vi "read.vi"() -> ()   [LabVIEW 2020]
panel:
  in  "lim 2":dbl
  in  "Temp":dbl(slide) scale=0.0..100.0
  out "Waveform Chart":dynamicdata(graph)
  in  "stop":bool
  out "alarma":bool
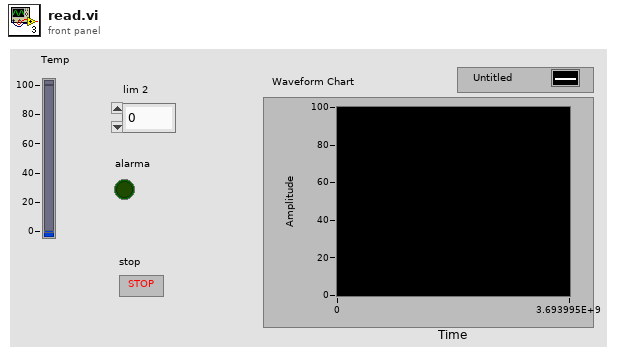
[diagram p1: front panel]
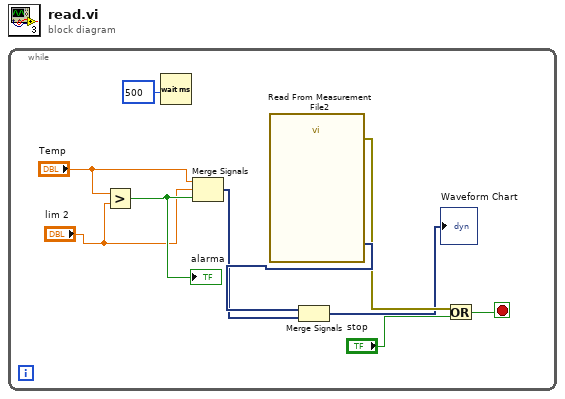
[diagram p0: block diagram]
diagram:
  n1 = while {
    stop <- w9 stop-if-true
    n2 = Greater?(x="Temp", y="lim 2") -> (0:w5:bool)
    "alarma" <- w5
    n3 = Wait (ms)(milliseconds to wait=500) -> ()  [unwired: 1 out]
    n4 = Merge Signals("Temp", "lim 2", w5) -> (w1:dynamicdata)
    n5 = call "Read From Measurement File2"() -> ("error out"=w6:errorcluster, "Signals"=w7:dynamicdata)  [unwired: 6 in, 4 out]
    n6 = Merge Signals(w7, w1) -> (→"Waveform Chart":dynamicdata)
    n7 = Or(x=w6, y="stop") -> (x .or. y?=w9:bool)
  }
